vi "temp_res_avg_block.vi"(9 "Avg":i32, 10 "Channel in":T1(ring), 11 "VISA Refnum in":refnum<visa-resource-name>) -> (2 "Numeric":dbl, 3 "Numeric 2":dbl)   [LabVIEW 2020]
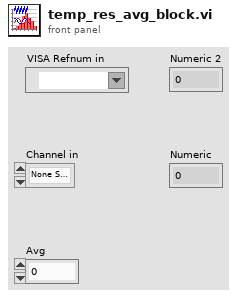
[diagram p1: front panel]
types:
  T1 = enum16{"None Selected", "1", "2", "3", "4", "5", "6", "7", "8", "9", "10", "11", "12", "13", "14", "15", "16"}
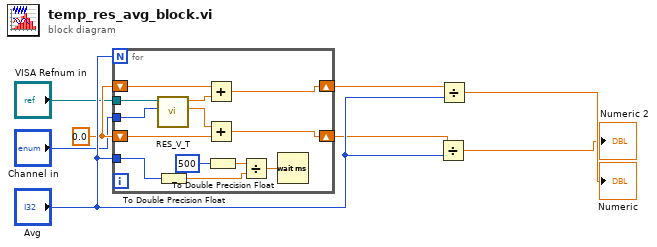
[diagram p0: block diagram]
diagram:
  w3 = 0.0
  n1 = for {
    N: "Avg" -> [_]
    tunnel: "Avg" -> [w17]
    tunnel: "VISA Refnum in" -> [w16]
    tunnel: "Channel in" -> [w15]
    shift-right: [w12] -> w4
    shift-left: w3 -> [w13]
    shift-right: [w9] -> w5
    shift-left: w3 -> [w11]
    n2 = call "RES_V_T.vi"("Channel"=w15, "VISA Refnum in"=w16) -> ("Numeric 2"=w10:dbl, "Numeric"=w14:dbl)  [unwired: 8 in]
    n3 = To Double Precision Float(number=w17) -> (double precision float=w19:dbl)
    n4 = Add(x=w13, y=w14) -> (x+y=w12:dbl)
    n5 = Add(x=w10, y=w11) -> (x+y=w9:dbl)
    n6 = To Double Precision Float(number=u32 500 ("milliseconds to wait")) -> (double precision float=w20:dbl)
    n7 = Divide(x=w20, y=w19) -> (x/y=w21:dbl)
    n8 = Wait (ms)(milliseconds to wait=w21) -> ()  [unwired: 1 out]
  }
  n9 = Divide(x=w5, y="Avg") -> (x/y=→"Numeric 2":dbl)
  n10 = Divide(x=w4, y="Avg") -> (x/y=→"Numeric":dbl)
